vi "AlarmLogic.vi"(0 "DSR":refnum<class "DataSocket Tag Reader.lvclass">, 1 "cfg":T1, 2 "ack":refnum<vi>) -> (14 "DSR out":refnum<class "DataSocket Tag Reader.lvclass">, 15 "AllarmeSuDO":bool)   [LabVIEW 2018]
uses:
  ControlCfg.ctl
  ControlConfigMisura.ctl
  ControlConfigDI.ctl
  <userlib>/ORI_DataSocketReader/DataSocket Tag Reader.lvclass
  <userlib>/ORI_DataSocketReader/Write Bool.vi
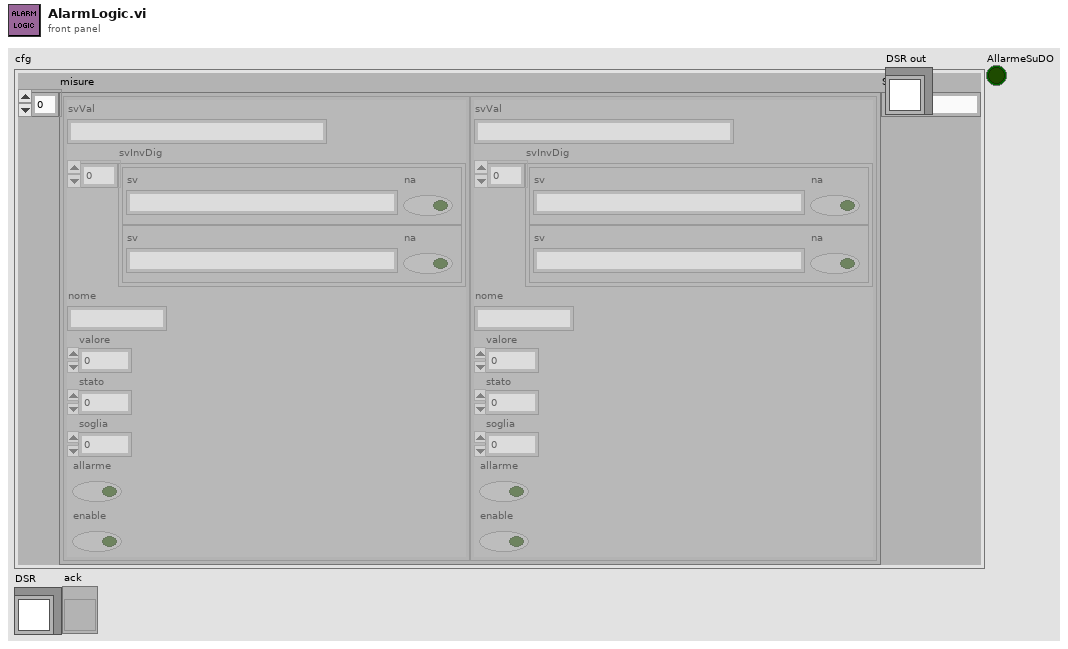
[diagram p1: front panel]
types:
  T1 = typedef "ControlCfg.ctl" = cluster{"misure":T2[], "SVDO":string}
  T2 = typedef "ControlConfigMisura.ctl" = cluster{"svVal":string, "svInvDig":T3[], "nome":string, "valore":dbl, "stato":i16, "soglia":dbl, "allarme":bool, "enable":bool}
  T3 = typedef "ControlConfigDI.ctl" = cluster{"sv":string, "na":bool}
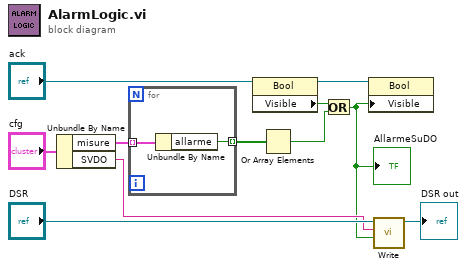
[diagram p0: block diagram]
diagram:
  n1 = Unbundle By Name("cfg") -> ("misure"=w10:T2[], "SVDO"=w3:string)
  n2 = for {
    tunnel: w10 -> [w13] mode=indexing
    tunnel: [w12] -> w6 mode=indexing
    n3 = Unbundle By Name(w13) -> ("allarme"=w12:bool)
  }
  n4 = property class="Bool"(reference="ack") -> (reference out=w2:refnum<vi>, "Visible"=w4:bool)  [unwired: 1 in, 1 out]
  n5 = Or Array Elements(Boolean array=w6) -> (logical OR=w5:bool)
  n6 = Or(x=w4, y=w5) -> (x .or. y?=w1:bool)
  "AllarmeSuDO" <- w1
  n7 = property class="Bool"(reference=w2, "Visible"=w1) -> ()  [unwired: 1 in, 2 out]
  n8 = call-poly <userlib>:"Write.vi"("Value"=w1, "tag"=w3, "DataSocket Tag Reader in"="DSR") -> ("DataSocket Tag Reader out"=→"DSR out":refnum<class "DataSocket Tag Reader.lvclass">)  [unwired: 5 in, 3 out]
